vi "FringeScanner-Idle.vi"(8 "error in (no error)":errorcluster) -> (0 "error out":errorcluster)   [LabVIEW 2009]
uses:
  Controls/FringeScannerCommand.ctl
  Controls/FringeScannerData.ctl
  Nicmos/Controls/NICMOS.READOUT.ctl
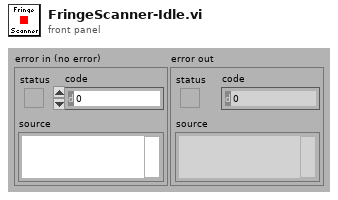
[diagram p1: front panel]
types:
  T1 = typedef "FringeScannerCommand.ctl" = cluster{"Command":enum16{"IDLE", "SCAN", "QUIT"}, "FringeScannerData":T2}
  T2 = typedef "FringeScannerData.ctl" = cluster{"Readout":T3, "Wavelength":dbl[unit], "Frame per fringe":dbl, "Autcollimation":bool}
  T3 = typedef "NICMOS.READOUT.ctl" = cluster{"Readout":i32, "Deglitch":i32, "Framerate":dbl[unit], "Bank":i32}
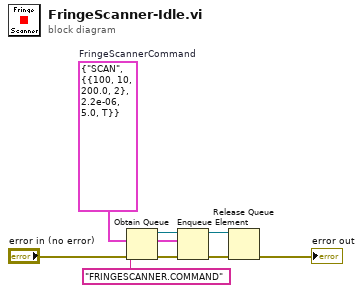
[diagram p0: block diagram]
diagram:
  w2 = T1 {"Command"=enum."SCAN", "FringeScannerData"={"Readout"={"Readout"=100, "Deglitch"=10, "Framerate"=200.0, "Bank"=2}, "Wavelength"=2.2e-06, "Frame per fringe"=5.0, "Autcollimation"=TRUE}}  # FringeScannerCommand
  n1 = Obtain Queue(name (unnamed)="FRINGESCANNER.COMMAND", element data type=w2, error in (no error)="error in (no error)") -> (queue out=w6:refnum<queue>, error out=w7:errorcluster)  [unwired: 2 in, 1 out]
  n2 = Enqueue Element(queue=w6, element=w2, error in (no error)=w7) -> (queue out=w5:refnum<queue>, error out=w4:errorcluster)  [unwired: 1 in, 1 out]
  n3 = Release Queue(queue=w5, error in (no error)=w4) -> (error out=→"error out":errorcluster)  [unwired: 1 in, 2 out]
